vi "Do.vi"(8 "error in (no error)":errorcluster, 10 "Actor in":refnum<class "Actor.lvclass">, 11 "Write DER SetpointVF Msg":refnum<class "Write DER SetpointF Msg.lvclass">) -> (0 "error out":errorcluster, 2 "Actor out":refnum<class "Actor.lvclass">)   [LabVIEW 2018, in "DER Actor.lvlib" / "Write DER SetpointF Msg.lvclass"]
doc: "This VI delivers the message to the actor by calling the appropriate method(s) on the actor."
uses:
  Write DER SetpointV Msg/Write DER SetpointF Msg.lvclass
  <vilib>/ActorFramework/Actor/Actor.lvclass
  DER/DER.lvclass
  C:/Program Files (x86)/National Instruments/LabVIEW 2018/vi.lib/ActorFramework/Actor/Actor.lvclass
  C:/Users/Administrator/Desktop/2018LabVIEW EMS/IED Actors/Device DDS Communications Framework/Device DDS Communications/Device DDS Communications.lvclass
  Write DER SetpointV Msg/Write DER SetpointF Msg.lvclass/Write DER SetpointF Msg.ctl
  Device DDS Communications Framework/Device DDS Communications/Device DDS Communications.lvclass/Device DDS Communications.ctl
  <vilib>/ORNL/CSEISMIC DDS/CSEISMIC DDS Base/CSEISMIC DDS.lvclass/CSEISMIC DDS.ctl
  Device DDS Communications Framework/Device DDS Communications/Accessors/Read DDS Writer Object.vi
  <vilib>/ORNL/CSEISMIC DDS/DDS Writer/Writers/Write DER_SetPointF.vi
  <vilib>/ORNL/CSEISMIC DDS/CSEISMIC DDS Base/Accessors/Read DDS Reference.vi
  <vilib>/ORNL/CSEISMIC DDS/DDS Writer/DDS Writer.lvclass
  C:/Program Files (x86)/National Instruments/LabVIEW 2018/vi.lib/ORNL/CSEISMIC DDS/CSEISMIC DDS Base/CSEISMIC DDS.lvclass
  <vilib>/ORNL/CSEISMIC DDS/CSEISMIC DDS Base/Error Handler.vi
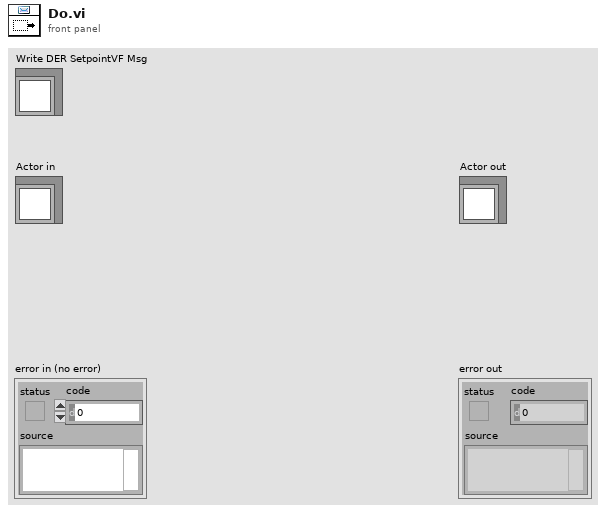
[diagram p1: front panel]
types:
  T1 = typedef "CSEISMIC DDS.lvlib/CSEISMIC DDS.lvclass/DER_SetPointF.ctl" = cluster{"DeviceID":T2, "Frequency (Hz)":dbl}
  T2 = typedef "CSEISMIC DDS.lvlib/CSEISMIC DDS.lvclass/DeviceID.ctl" = string
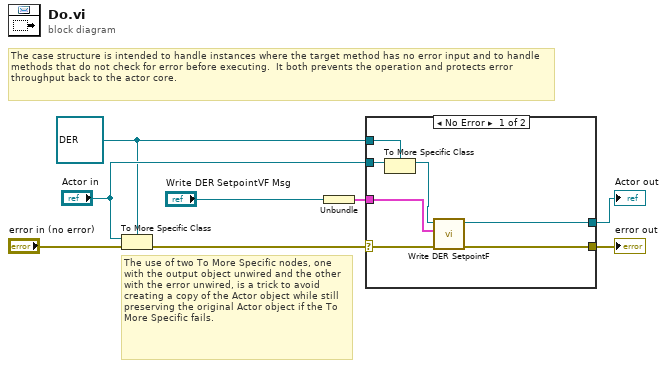
[diagram p0: block diagram]
diagram:
  w2 = refnum<class "DER.lvclass"> refnum ("Actor in")
  # "The use of two To More Specific nodes, one with the output object unwired and the other with the error unwired, is a trick to avoid creating a copy of the Actor object while still preserving the original Actor object if the To More Specific fails."
  # "The case structure is intended to handle instances where the target method has no error input and to handle methods that do not check for error before executing.  It both prevents the operation and protects error throughput back to the actor core."
  n1 = To More Specific Class(target class=w2, reference="Actor in", error in="error in (no error)") -> (error out=w6:errorcluster)  [unwired: 1 out]
  n2 = Unbundle("Write DER SetpointVF Msg") -> (w1:T1)
  n3 = case shown="No Error" w6 {
    selector: w6 -> [w11 w17]
    tunnel: [w12 w17] -> w5
    tunnel: [w13 w16] -> w4
    tunnel: "Actor in" -> [w15 w16]
    tunnel: w2 -> [w14 _]
    tunnel: w1 -> [w10 _]
    frame No Error {
      n4 = To More Specific Class(target class=w14, reference=w15) -> (specific class reference=w9:refnum<class "DER.lvclass">)  [unwired: 1 in, 1 out]
      n5 = call "Write DER SetpointF.vi"("error in"=w11, "DER_SetPointF"=w10, "DER in"=w9) -> ("error out"=w12:errorcluster, "DER out"=w13:refnum<class "DER.lvclass">)  [unwired: 7 in]
    }
    frame Error {
      # "If type check fails, pass the original object out again."
    }
  }
  "error out" <- w5
  "Actor out" <- w4
